vi "NUM U8_ASCII (SubVI).vi"(1 "Numeric":i32) -> (0 "String out":string)   [LabVIEW 8.6]
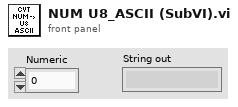
[diagram p1: front panel]
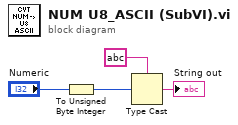
[diagram p0: block diagram]
diagram:
  n1 = To Unsigned Byte Integer(number="Numeric") -> (unsigned 8bit integer=w3:u8)
  n2 = Type Cast(type=string ?, x=w3) -> (*(type *) &x=→"String out":string)
